vi "SV Power Spectrum Info Probe.vi"(1 "spectrum info":T2 {"x-axis units" items=["Time (s)"=0, "Frequency-CB (Hz)"=1, "Frequency-CPB (Hz)"=1248, "Frequency-Arbitrary (Hz)"=2357, "Quefrency (s)"=2, "Revolutions (rev)"=3, "Order"=4, "Speed (RPM)"=11, "Speed (rad/s)"=21, "Index"=65535]; "weighting filter" items=["Linear", "A-weighting", "B-weighting", "C-weighting", "ITU-R 468-4", "Dolby", "CCITT", "C-message", "Wb", "Wc", "Wd", "We", "Wf", "Wh", "Wj", "Wk", "Wm", "AES17 20 kHz lowpass", "AES17 40 kHz lowpass", "AES17 20 kHz highpass", "AES17 40 kHz highpass"]; "dB reference [EU]" format="%.2f"; "engineering units" items=["custom..."=0, "V"=1, "A"=21, "C"=30, "pC"=31, "s"=32, "-"=29, "Pa"=2, "N"=20, "g"=3, "m/s^2"=4, "m/s"=5, "m"=6, "mm/s"=12, "mm"=13, "micron/s"=14, "micron"=15, "in/s^2"=7, "in/s"=8, "in"=9, "mil/s"=10, "mil"=11, "rad/s^2"=16, "rad/s"=17, "rad"=18, "deg/s^2"=26, "deg/s"=27, "deg"=28, "RPM"=22, "cycle/s^2"=23, "Hz"=24, "cycle"=25, "strain"=19]; "spectral info"."window" items=["None "=0, "Hanning"=1, "Hamming"=2, "Blackman-Harris"=3, "Exact Blackman"=4, "Blackman"=5, "Flat Top"=6, "4 Term B-Harris "=7, "7 Term B-Harris"=8, "Low Sidelobe"=9, "Force - Exponential"=10, "Gaussian"=62]}) -> (0 "Boolean":bool)   [LabVIEW 2017]
uses:
  <vilib>/addons/_NISVFA/_Shared subVIs/Controls/svc_Spectrum Info.ctl
  <vilib>/addons/_NISVFA/_Shared subVIs/Controls/svc_X-Axis Units.ctl
  <vilib>/addons/_NISVFA/_Shared subVIs/Controls/svc_Spectrum Type.ctl
  <vilib>/addons/_NISVFA/_Shared subVIs/Controls/svc_Engineering Units Text Ring.ctl
  <vilib>/addons/_NISVFA/_Shared subVIs/Controls/svc_Weighting Filter Text Ring.ctl
  <vilib>/addons/_NISVFA/_Shared subVIs/Controls/svc_Complimentary Spectrum Units.ctl
  <vilib>/addons/_NISVFA/_Shared subVIs/Controls/NI Spectrum Component.ctl
panel:
  out "y-axis label":string
  out "x-axis unit label":string
  out "window parameter":dbl format="%.2f"
  out "spectrum skewed":bool
  out "spectral density":bool
  out "x-axis label":string
  out "peak units":enum16{"rms", "peak", "peak-peak"}(ring)
  out "weighting filter":u16(ring) items=["Linear", "A-weighting", "B-weighting", "C-weighting", "ITU-R 468-4", "Dolby", "CCITT", "C-message"]
  out "custom label":string
  out "dB reference [EU]":dbl format="%#_3p"
  out "engineering units":u16(ring) items=["custom..."=0, "V"=1, "A"=21, "Pa"=2, "N"=20, "g"=3, "m/s^2"=4, "m/s"=5, "m"=6, "mm/s"=12, "mm"=13, "microns/s"=14, "microns"=15, "in/s^2"=7, "in/s"=8, "in"=9, "mils/s"=10, "mils"=11, "rad/s^2"=16, "rad/s"=17, "rad"=18, "strain"=19]
  out "FFT size":i32
  out "window size":i32
  out "window":u16(ring) items=["None "=0, "Hanning"=1, "Hamming"=2, "Blackman-Harris"=3, "Exact Blackman"=4, "Blackman"=5, "Flat Top"=6, "4 Term B-Harris "=7, "7 Term B-Harris"=8, "Low Sidelobe"=9, "Force - Exponential"=10, "Gaussian"=62]
  out "linear/dB":enum16{"linear", "dB"}(ring)
  out "spectrum type":T1(ring)
  out "y-axis unit label":string
  out "description":string
  out "channel name":string
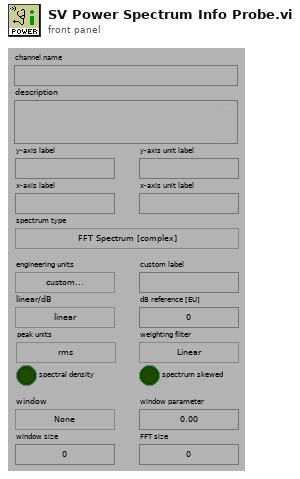
[diagram p1: front panel]
types:
  T1 = enum16{"FFT Spectrum [complex]", "Amplitude [Magnitude]", "Power [Magnitude^2]", "Cross Spectrum [complex]", "Frequency Response [Complex]"}
  T2 = typedef "svc_Spectrum Info.ctl" = cluster{"channel name":string, "description":string, "x-axis units":T3, "spectral info":cluster{"spectrum type":T4, "linear/dB":enum16{"linear", "dB"}, "window":u16, "window size":i32, "FFT size":i32}, "engineering units":T5, "custom label":string, "dB reference [EU]":dbl, "peak units":enum16{"rms", "peak", "peak-peak"}, "weighting filter":T6, "spectral density?":bool, "unit label":string, "spectrum skewed?":bool, "complimentary spectrum units":T7}
  T3 = typedef "svc_X-Axis Units.ctl" = u16
  T4 = typedef "svc_Spectrum Type.ctl" = enum16{"FFT Spectrum [complex]", "Amplitude [Magnitude]", "Power [Magnitude^2]", "Cross Spectrum [complex]", "Frequency Response [Complex]"}
  T5 = typedef "svc_Engineering Units Text Ring.ctl" = u16
  T6 = typedef "svc_Weighting Filter Text Ring.ctl" = u16
  T7 = typedef "svc_Complimentary Spectrum Units.ctl" = enum16{"none", "radians", "degrees", "cycles", "imaginary"}
  T8 = typedef "NI Spectrum Component.ctl" = u16
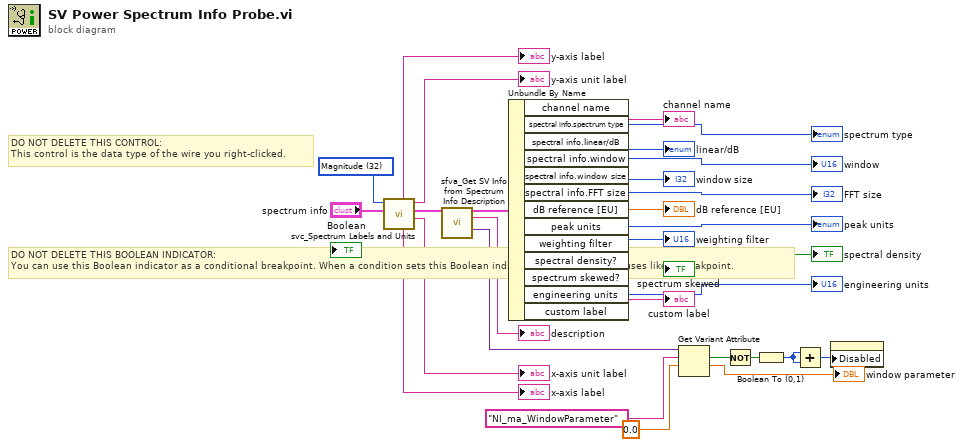
[diagram p0: block diagram]
diagram:
  w25 = T8 32 items=["Magnitude"=32, "Phase"=33, "Real"=34, "Imaginary"=35, "Coherence"=36, "Unknown"=99] ("spectrum component")
  # "DO NOT DELETE THIS BOOLEAN INDICATOR: \nYou can use this Boolean indicator as a conditional breakpoint. When a condition sets this Boolean indicator to TRUE, the VI pauses like a breakpoint."
  # "DO NOT DELETE THIS CONTROL: \nThis control is the data type of the wire you right-clicked."
  n1 = call <vilib>:"svc_Spectrum Labels and Units.vi"("spectrum info in"="spectrum info", "spectrum component"=w25) -> ("x-axis unit label"=→"x-axis unit label":string, "spectrum info out"=w29:T2, "unit label"=→"y-axis unit label":string, "x-axis label"=→"x-axis label":string, "y-axis label"=→"y-axis label":string)  [unwired: 4 in, 1 out]
  n2 = call <vilib>:"sfva_Get SV Info from Spectrum Info Description.vi"("spectrum info"=w29) -> ("spectrum info"=w22:T2, "description"=→"description":string, "SV Info"=w6:variant)  [unwired: 10 in, 2 out]
  n3 = Unbundle By Name(w22) -> ("channel name"=→"channel name":string, "spectral info.spectrum type"=→"spectrum type":T4, "spectral info.linear/dB"=→"linear/dB":enum16{"linear", "dB"}, "spectral info.window"=→"window":u16, "spectral info.window size"=→"window size":i32, "spectral info.FFT size"=→"FFT size":i32, "dB reference [EU]"=→"dB reference [EU]":dbl, "peak units"=→"peak units":enum16{"rms", "peak", "peak-peak"}, "weighting filter"=→"weighting filter":T6, "spectral density?"=→"spectral density":bool, "spectrum skewed?"=→"spectrum skewed":bool, "engineering units"=→"engineering units":T5, "custom label"=→"custom label":string)
  n4 = Get Variant Attribute(Variant=w6, name="NI_ma_WindowParameter", default value (empty Variant)=0.0 ("window parameter")) -> (found=w4:bool, value=→"window parameter":dbl)  [unwired: 1 in, 2 out]
  n5 = Not(x=w4) -> (.not. x?=w1:bool)
  n6 = Boolean To (0,1)(Boolean=w1) -> (0, 1=w3:i16)
  n7 = Add(x=w3, y=w3) -> (x+y=w2:i16)
  n8 = property on="window parameter" class="DigNum (strict)"("Disabled"=w2) -> ()  [unwired: 2 in, 2 out]
